vi "Write ResponseHeader.vi"(8 "error in (no error)":errorcluster, 10 "LabVIEWHTTPClient_NET.lvlib:HttpHeaders_Response.lvclass":refnum<class "HttpHeaders_Response.lvclass">, 11 "REST Client Headers_NET in":refnum<class "REST Client Headers_NET.lvclass">) -> (0 "error out":errorcluster, 3 "REST Client Headers_NET out":refnum<class "REST Client Headers_NET.lvclass">)   [LabVIEW 2018, in "REST Client_NET.lvlib" / "REST Client Headers_NET.lvclass"]
doc: "<b> </b> <b> </b>\nHttpClient_NET\nJustin Young - Viviota\nCopyright (c) 2021\nLicense: BSD"
uses:
  REST Client Headers_NET.lvclass
  HttpHeaders_response/HttpHeaders_Response.lvclass
  REST Client Headers_NET.lvclass/REST Client Headers_NET.ctl
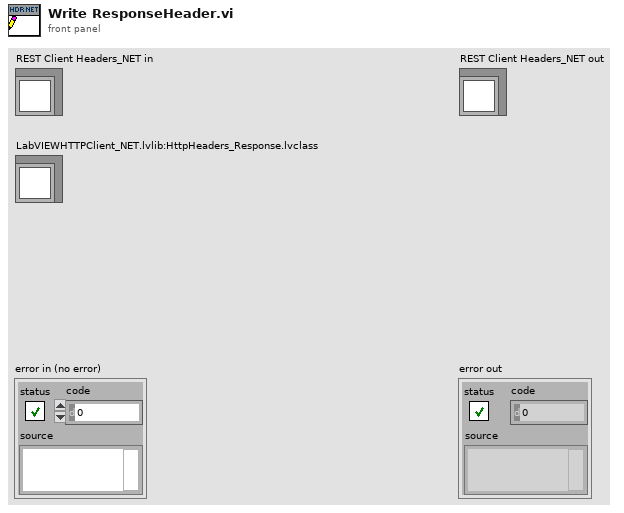
[diagram p1: front panel]
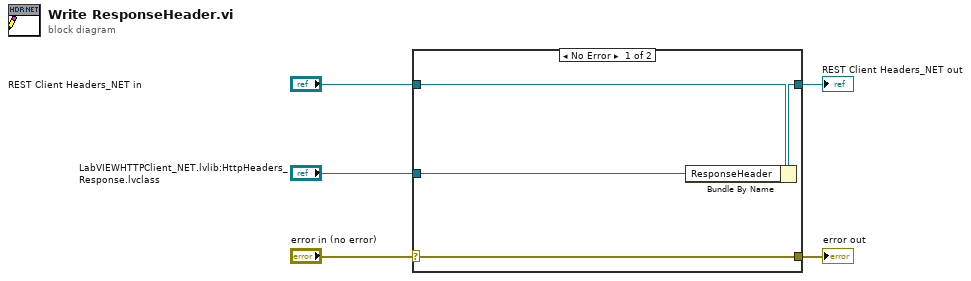
[diagram p0: block diagram]
diagram:
  n1 = case shown="No Error" "error in (no error)" {
    selector: "error in (no error)" -> [w9 w10]
    tunnel: [w9 w10] -> w4
    tunnel: [w7 w11] -> w2
    tunnel: "REST Client Headers_NET in" -> [w8 w11]
    tunnel: "LabVIEWHTTPClient_NET.lvlib:HttpHeaders_Response.lvclass" -> [w6 _]
    frame No Error {
      n2 = Bundle By Name(cluster=w8, "ResponseHeader"=w6) -> (w7:refnum<class "REST Client Headers_NET.lvclass">)
    }
    frame Error {
    }
  }
  "error out" <- w4
  "REST Client Headers_NET out" <- w2
